vi "ad stop scan.vi"(8 "error in (no error)":errorcluster, 10 "result":i32[](array[numeric]), 11 "adh":i32) -> (0 "error out":errorcluster, 2 "function return":i32, 3 "result out":i32[](array[numeric]))   [LabVIEW 2021, in "libad4.lvlib"]
doc: "ad_stop_scan (int32_t adh, int32_t *result);\n\nStops a continuous or memory scan. Any scan that has been started successfully must be stopped with ad_stop_scan."
uses:
  <userlib>/libad4/libad4.lvlib
  <userlib>/libad4/libad4.dll
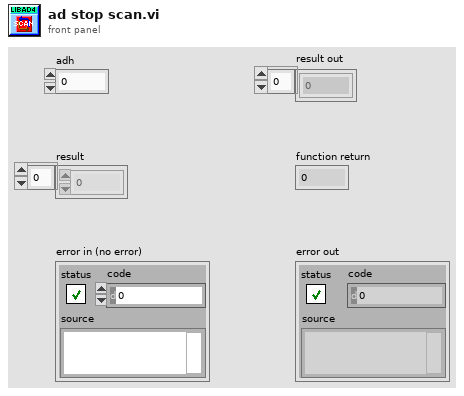
[diagram p1: front panel]
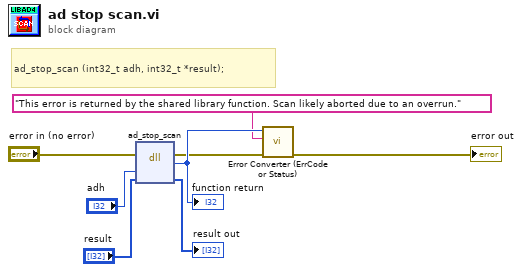
[diagram p0: block diagram]
diagram:
  # "ad_stop_scan (int32_t adh, int32_t *result);"
  n1 = dll-call lib="C:/Program Files/National Instruments/LabVIEW 2021/user.lib/libad4/libad4.*" fn="ad_stop_scan"(error in="error in (no error)", "adh"="adh", "result"="result") -> (error out=w5:errorcluster, "return type"=w8:i32, "result"=→"result out":i32[])  [unwired: 3 in, 1 out]
  "function return" <- w8
  n2 = call <userlib>:"Error Converter (ErrCode or Status).vi"("error in (no error)"=w5, "string"="This error is returned by the shared library function. Scan likely aborted due to an overrun.", "error code"=w8) -> ("error out"=→"error out":errorcluster)  [unwired: 8 in]
